vi "Drive Cycle Engine Request State ERD.vi"(0 "GEA2 Reference In":refnum<k24>, 1 "GEA Inputs":T2 {"Destination" format="%.0x"; "Source" format="%.0x"}, 2 "Standalone?":bool, 7 "Cycle ID":u8, 9 "Drive Cycle Engine Request State":T1=enum."Select", 11 "Error In":errorcluster) -> (4 "GEA2 Reference Out":refnum<k24>, 15 "Error Out":errorcluster)   [LabVIEW 2016, in "TL27.lvlib"]
doc: "This vi can be used to update the MC cycle engine state with the requested values."
uses:
  Projects/TL27.lvlib
  C:/Automation/DLLs/PC Dot Net/GeaCommunication.dll
  Common/LabVIEW GEA2 Toolkit/LabVIEW_GEA2_Toolkit.lvlibp/type defs/Source_Destination.ctl
  type defs/Drive Cycle Engine Request State.ctl
  Common/LabVIEW GEA2 Toolkit/LabVIEW_GEA2_Toolkit.lvlibp/type defs/ERD Write Data In.ctl
  Common/LabVIEW GEA2 Toolkit/LabVIEW_GEA2_Toolkit.lvlibp/type defs/Data Type.ctl
  Common/LabVIEW GEA2 Toolkit/LabVIEW_GEA2_Toolkit.lvlibp
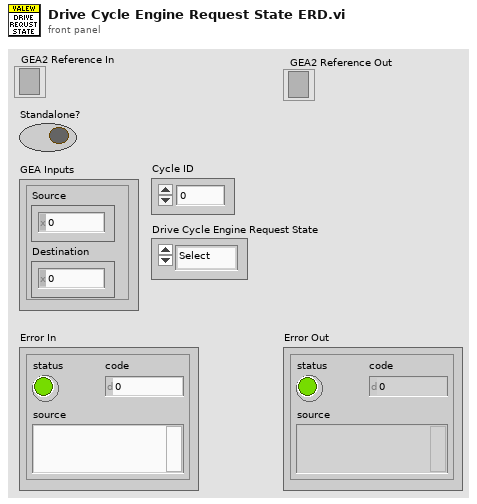
[diagram p1: front panel]
types:
  T1 = typedef "TL27.lvlib/Drive Cycle Engine Request State.ctl" = enum16{"Start", "Stop", "Pause", "Resume", "Select"}
  T2 = typedef "LabVIEW_GEA2_Toolkit.lvlibp/Source_Destination.ctl" = cluster{"Source":u8, "Destination":u8}
  T3 = typedef "LabVIEW_GEA2_Toolkit.lvlibp/ERD Write Data In.ctl" = cluster{"ERD Number":u16, "Data Type":T4, "Data":string}
  T4 = typedef "LabVIEW_GEA2_Toolkit.lvlibp/Data Type.ctl" = enum16{"string", "boolean", "uint8_t", "uint16_t", "uint32_t", "uint64_t", "int8_t", "int16_t", "int32_t", "int64_t"}
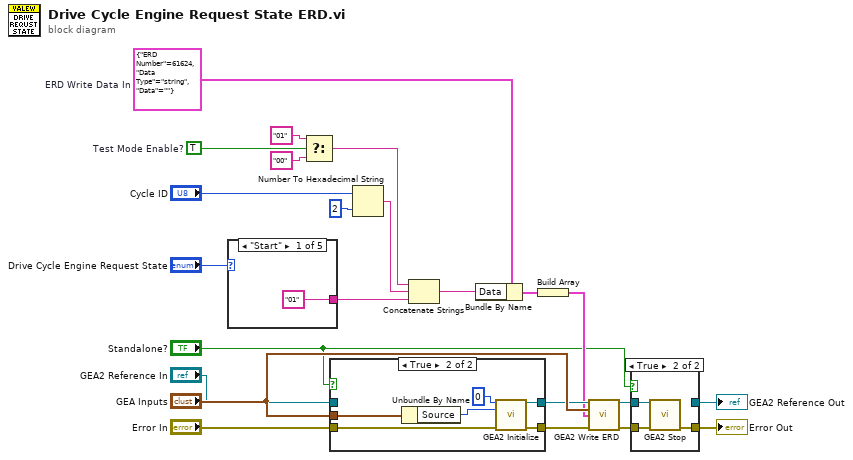
[diagram p0: block diagram]
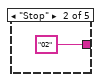
[diagram p2: hidden frame]
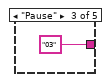
[diagram p3: hidden frame]
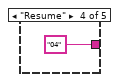
[diagram p4: hidden frame]
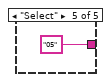
[diagram p5: hidden frame]
diagram:
  w5 = TRUE  # Test Mode Enable?
  w22 = T3 {"ERD Number"=61624, "Data Type"=enum."string", "Data"=""}  # ERD Write Data In
  n1 = case shown="\"Start\"" "Drive Cycle Engine Request State" {
    tunnel: ["01" ("Message") "02" ("Message") "03" ("Message") "04" ("Message") "05" ("Message")] -> w6
    frame "Start" {
    }
    frame "Stop" {
    }
    frame "Pause" {
    }
    frame "Resume" {
    }
    frame "Select" {
    }
  }
  n2 = Select(t="01" ("Message"), s=w5, f="00" ("Message")) -> (s? t:f=w8:string)
  n3 = case shown="True" "Standalone?" {
    tunnel: "Error In" -> [w29 w36]
    tunnel: [w29 w35] -> w3
    tunnel: "GEA2 Reference In" -> [w30 _]
    tunnel: [w30 w34] -> w19
    tunnel: "GEA Inputs" -> [_ w32]
    frame False {
    }
    frame True {
      n4 = Unbundle By Name(w32) -> ("Source"=w33:u8)
      n5 = call "GEA2 Initialize.vi"("Board Index"=0, "Source Address"=w33, "error in"=w36) -> ("GEA2 Reference Out"=w34:refnum<k24>, "error out"=w35:errorcluster)  [unwired: 10 in, 1 out]
    }
  }
  n6 = Number To Hexadecimal String(1:i16 2 ("width (-)"), 2:"Cycle ID") -> (0:w7:string)
  n7 = Concatenate Strings(w8, w7, w6) -> (w1:string)
  n8 = Bundle By Name(cluster=w22, "Data"=w1) -> (w17:T3)
  n9 = Build Array(w17) -> (w18:T3[])
  n10 = call "GEA2 Write ERD.vi"("GEA2 Reference In"=w19, "GEA Inputs"="GEA Inputs", "Write ERD List"=w18, "Error In"=w3) -> ("GEA2 Reference Out"=w20:refnum<k24>, "Error Out"=w21:errorcluster)  [unwired: 9 in, 1 out]
  n11 = case shown="True" "Standalone?" {
    tunnel: w21 -> [w37 w41]
    tunnel: [w37 w40] -> w16
    tunnel: w20 -> [w38 w39]
    tunnel: [w38 _] -> w15
    frame False {
    }
    frame True {
      n12 = call "GEA2 Stop.vi"("GEA2 Reference In"=w39, "Error In"=w41) -> ("Error Out"=w40:errorcluster)  [unwired: 13 in]
    }
  }
  "Error Out" <- w16
  "GEA2 Reference Out" <- w15
